vi "Read Control Label.vi"(8 "error in (no error)":errorcluster, 11 "ControlMouseLeaveMsg in":refnum<class "ControlMouseLeaveMsg.lvclass">) -> (0 "error out":errorcluster, 2 "Control Label":string, 3 "ControlMouseLeaveMsg out":refnum<class "ControlMouseLeaveMsg.lvclass">)   [LabVIEW 2017, in "ActorEvents.lvlib" / "ControlMouseLeaveMsg.lvclass"]
uses:
  ControlMouseLeaveMsg.lvclass
  ControlMouseLeaveMsg.lvclass/ControlMouseLeaveMsg.ctl
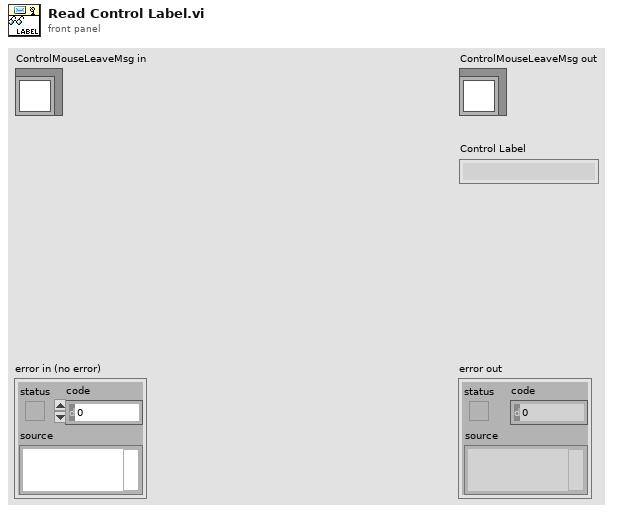
[diagram p1: front panel]
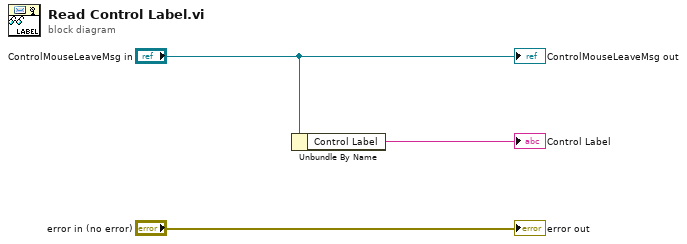
[diagram p0: block diagram]
diagram:
  n1 = Unbundle By Name("ControlMouseLeaveMsg in") -> ("Control Label"=→"Control Label":string)
  "error out" <- "error in (no error)"
  "ControlMouseLeaveMsg out" <- "ControlMouseLeaveMsg in"
